vi "AM Cycle CW.vi"(8 "error in (no error)":errorcluster, 10 "Message Queues in":T1, 11 "Data Cluster":T2 {"PS Measure Plan" items=["Pretreatment settings (PS)", "Linear Sweep Voltammetry (LSV)", "Differential Pulse Voltammetry (DPV)", "Cyclic Voltammetry (CV)", "Chronoamperometry (CA)", "Chronopotentiometry (CP)", "El Imp Spectroscopy (EIS)"]; "System Preset"."Test Configuration"."SP List" format="%#.1g"}) -> (0 "error out":errorcluster, 3 "Data Cluster out":T2 {"PS Measure Plan" items=["Pretreatment settings (PS)", "Linear Sweep Voltammetry (LSV)", "Differential Pulse Voltammetry (DPV)", "Cyclic Voltammetry (CV)", "Chronoamperometry (CA)", "Chronopotentiometry (CP)", "El Imp Spectroscopy (EIS)"]; "System Preset"."Test Configuration"."SP List" format="%#.1g"})   [LabVIEW 2020, in "Test Driver.lvlib"]
uses:
  Test Driver.lvlib
  Test Driver Configuration.ctl
  support/Message Queue/Message Cluster.ctl
  System Preset.ctl
  Test Type.ctl
  support/Message Queue/All Message Queues.ctl
  support/Message Queue/Message Queue.lvlib
panel:
  # "X"
  # "Y"
  # "Cycles"
  # "Point Delay"
  # "Up"
  # "Down"
  # "Z Axes"
  # "#C"
  # "In"
  # "Out"
  # "Cleaning [sec]"
  # "X"
  # "Y"
  # "Cycles"
  # "Point Delay"
  # "Up"
  # "Down"
  # "Z Axes"
  # "#C"
  # "In"
  # "Out"
  # "Cleaning [sec]"
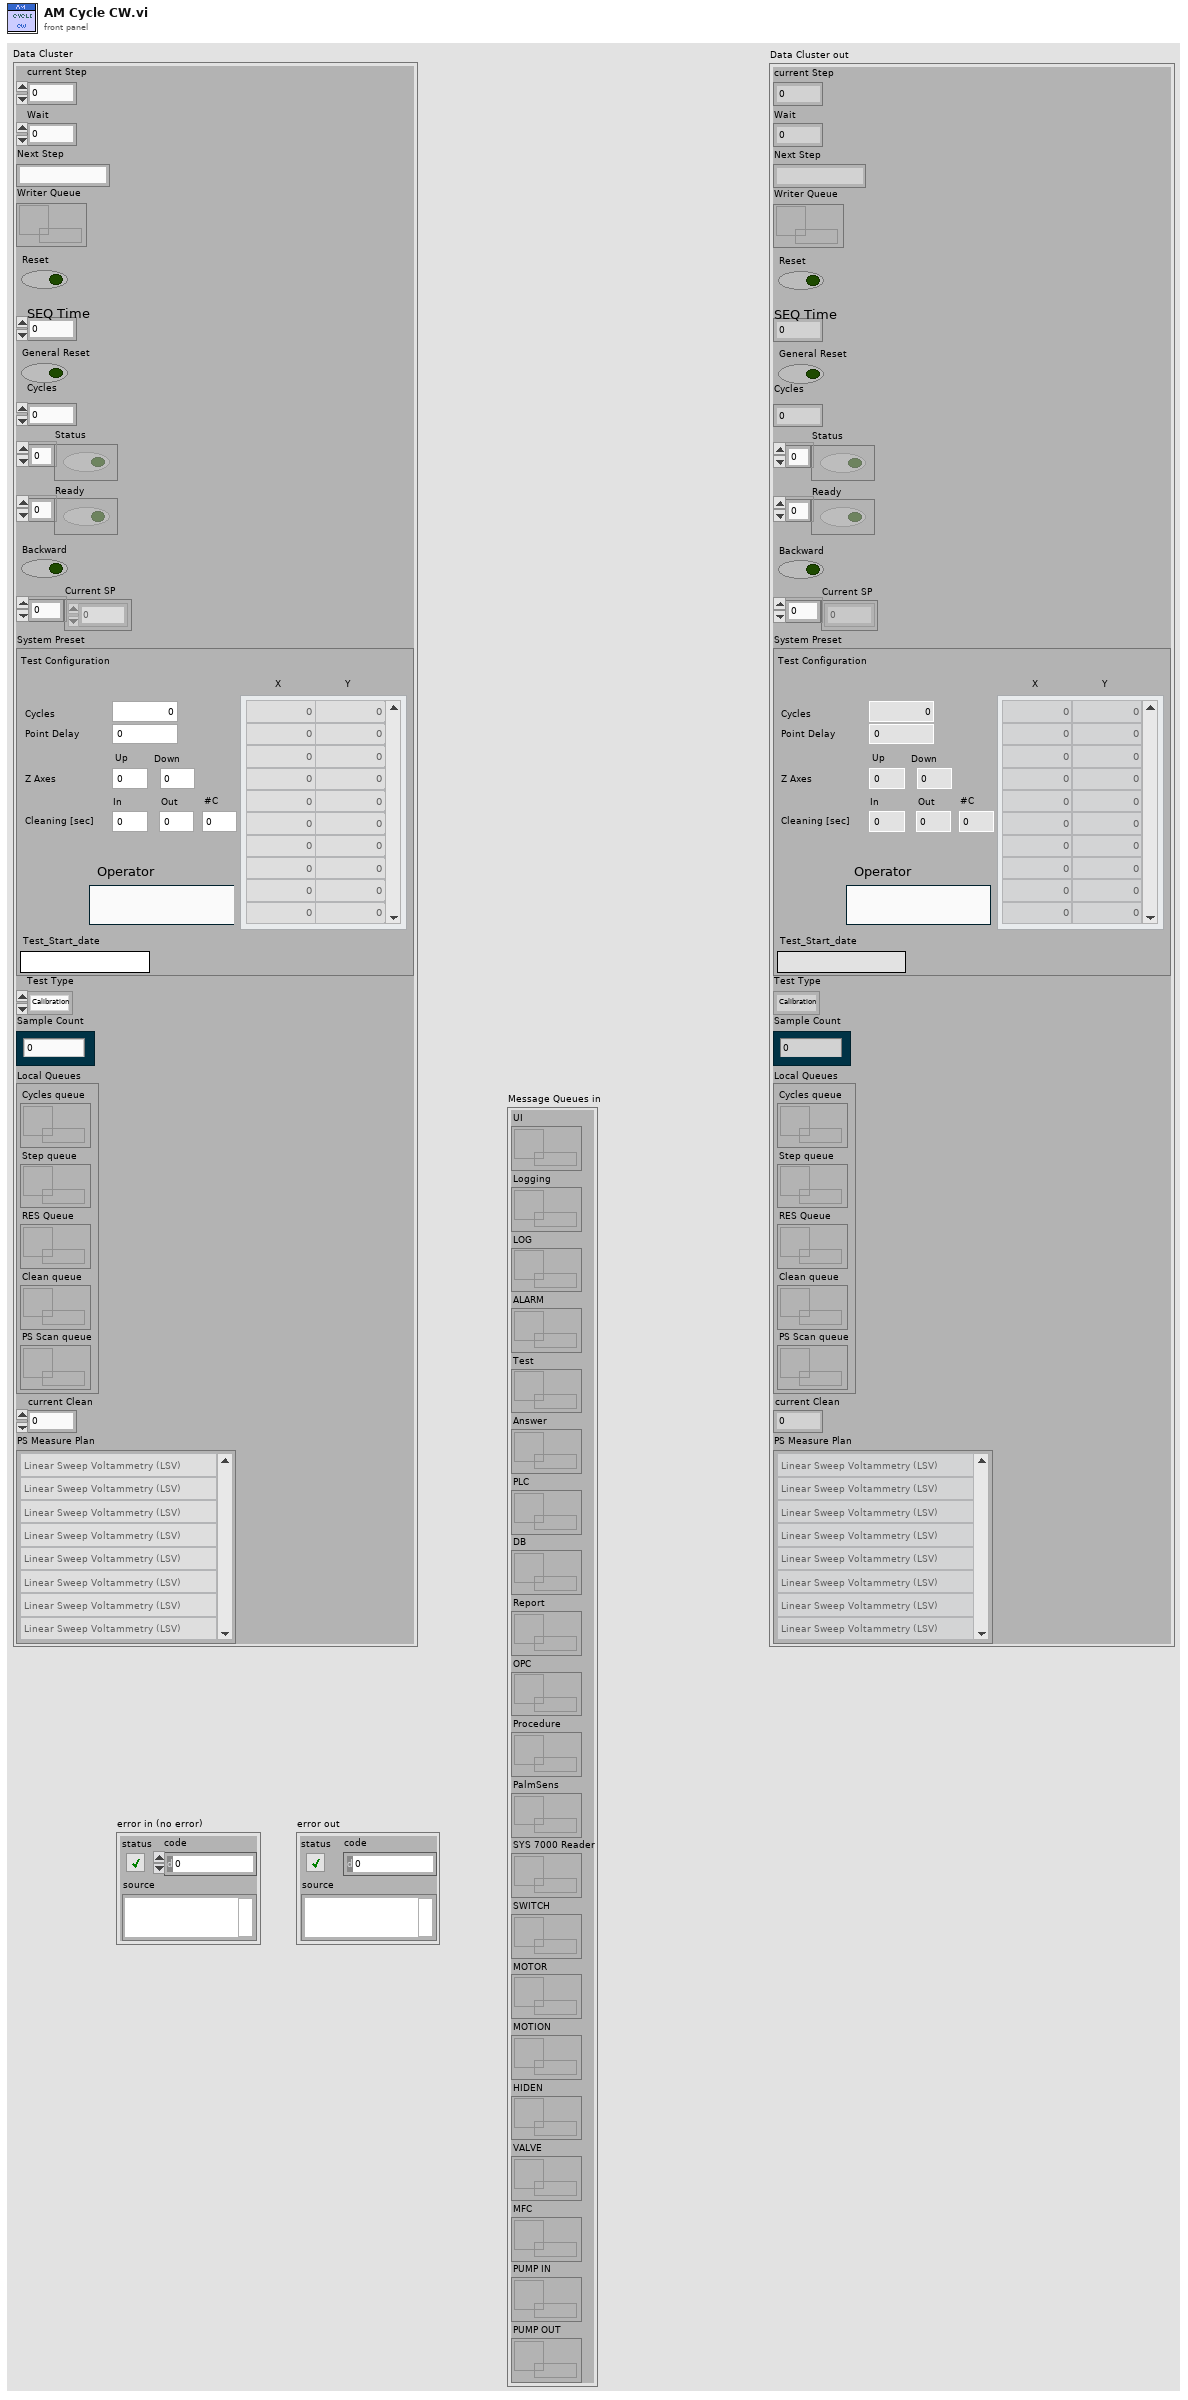
[diagram p1: front panel]
types:
  T1 = typedef "Message Queue.lvlib/All Message Queues.ctl" = cluster{"UI":refnum<queue>, "Logging":refnum<queue>, "LOG":refnum<queue>, "ALARM":refnum<queue>, "Test":refnum<queue>, "Answer":refnum<queue>, "PLC":refnum<queue>, "DB":refnum<queue>, "Report":refnum<queue>, "OPC":refnum<queue>, "Procedure":refnum<queue>, "PalmSens":refnum<queue>, "SYS 7000 Reader":refnum<queue>, "SWITCH":refnum<queue>, "MOTOR":refnum<queue>, "MOTION":refnum<queue>, "HIDEN":refnum<queue>, "VALVE":refnum<queue>, "MFC":refnum<queue>, "PUMP IN":refnum<queue>, "PUMP OUT":refnum<queue>}
  T2 = typedef "Test Driver.lvlib/Test Driver Configuration.ctl" = cluster{"current Step":i32, "Wait":dbl, "Next Step":string, "Writer Queue":refnum<queue>, "Reset":bool, "SEQ Time":i32, "General Reset":bool, "Cycles":i32, "Status":bool[], "Ready":bool[], "Backward":bool, "Current SP":dbl[], "System Preset":T3, "Test Type":T4, "Sample Count":i32, "Local Queues":cluster{"Cycles queue":refnum<queue>, "Step queue":refnum<queue>, "RES Queue":refnum<queue>, "Clean queue":refnum<queue>, "PS Scan queue":refnum<queue>}, "current Clean":i32, "PS Measure Plan":u16[]}
  T3 = typedef "System Preset.ctl" = cluster{"Test Configuration":cluster{"Cycles":i32, "Z Up":dbl, "SP List":dbl[][], "Operator":string, "Point Delay":i32, "Z Up 2":dbl, "Cleaning In":dbl, "Cleaning Out":dbl, "Cleaning Cycles":i32}, "Test_Start_date":string}
  T4 = typedef "Test Driver.lvlib/Test Type.ctl" = enum16{"Calibration", "Test"}
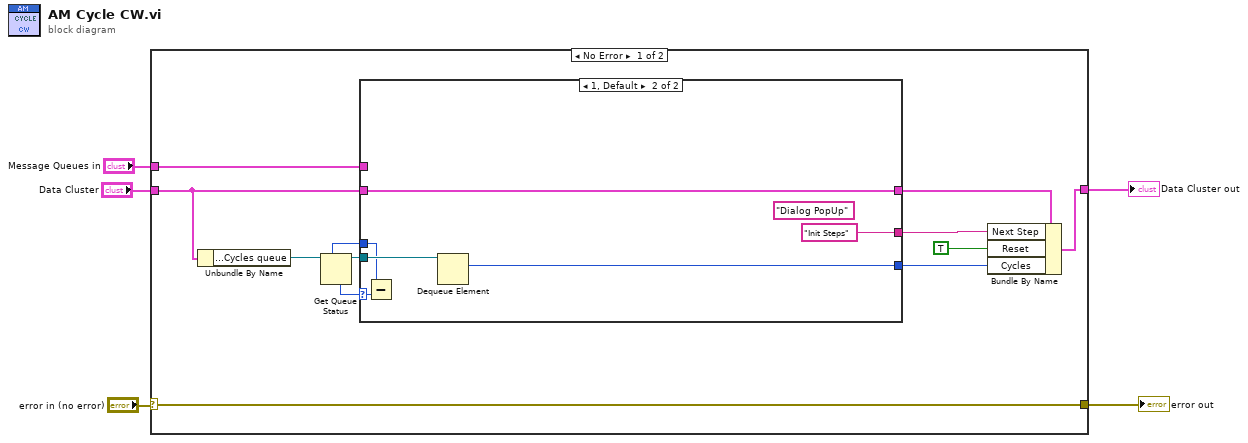
[diagram p0: block diagram]
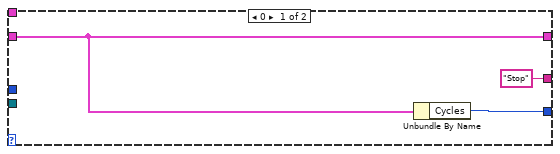
[diagram p2: hidden frame]
diagram:
  n1 = case shown="No Error" "error in (no error)" {
    selector: "error in (no error)" -> [w17 w27]
    tunnel: [w12 w28] -> w4
    tunnel: "Data Cluster" -> [w14 w28]
    tunnel: [w17 w27] -> w3
    tunnel: "Message Queues in" -> [w7 _]
    frame No Error {
      n2 = Unbundle By Name(w14) -> ("Local Queues.Cycles queue"=w16:refnum<queue>)
      n3 = Get Queue Status(queue=w16) -> (queue out=w15:refnum<queue>, max queue size=w8:i32, # elements in queue=w9:i32)  [unwired: 2 in, 5 out]
      n4 = case shown="1, Default" w9 {
        selector: w9 -> [_ w24]
        tunnel: w15 -> [_ w26]
        tunnel: [w19 w23] -> w13
        tunnel: w14 -> [w19 w23]
        tunnel: ["Stop" "Init Steps" ("Message")] -> w11
        tunnel: w7 -> [_ _]
        tunnel: w8 -> [_ w25]
        tunnel: [w18 w22] -> w6
        frame 0 {
          n5 = Unbundle By Name(w19) -> ("Cycles"=w18:i32)
        }
        frame 1, Default {
          (unwired) "Dialog PopUp" ("Message")
          n6 = Subtract(x=w25, y=w24) -> ()  [unwired: 1 out]
          n7 = Dequeue Element(queue=w26) -> (element=w22:i32)  [unwired: 2 in, 3 out]
        }
      }
      n8 = Bundle By Name(cluster=w13, "Next Step"=w11, "Reset"=TRUE, "Cycles"=w6) -> (w12:T2)
    }
    frame Error {
    }
  }
  "error out" <- w3
  "Data Cluster out" <- w4
